vi "URG-04LX-UG01 Start Acquisition.vi"(8 "VISA Refnum in 2":refnum<visa-resource-name>, 10 "Acquisition Parameters":T1={"Starting Step"=0, "Ending Step"=0, "Cluster Count"=0, "Scan Interval"=0, "Number of Scans"=0, "Measurement Type"=enum."MS"}, 11 "error in (no error)":errorcluster) -> (0 "VISA Refnum in":refnum<visa-resource-name>, 2 "Acquisition Parameters":T1={"Starting Step"=0, "Ending Step"=0, "Cluster Count"=0, "Scan Interval"=0, "Number of Scans"=0, "Measurement Type"=enum."MS"}, 3 "error out":errorcluster)   [LabVIEW 2018]
doc: "Begins an acquisition task with the URG-04LX-UG01 based upon the specified <b>Acquisition Parameters</b>."
uses:
  Type Definitions/Acquisition Parameters.ctl
  Type Definitions/Measurement Type.ctl
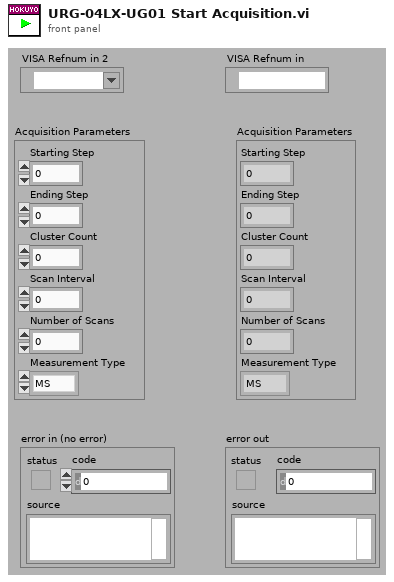
[diagram p1: front panel]
types:
  T1 = typedef "Acquisition Parameters.ctl" = cluster{"Starting Step":i32, "Ending Step":i32, "Cluster Count":i32, "Scan Interval":i32, "Number of Scans":i32, "Measurement Type":T2}
  T2 = typedef "Measurement Type.ctl" = enum16{"MD", "MS"}
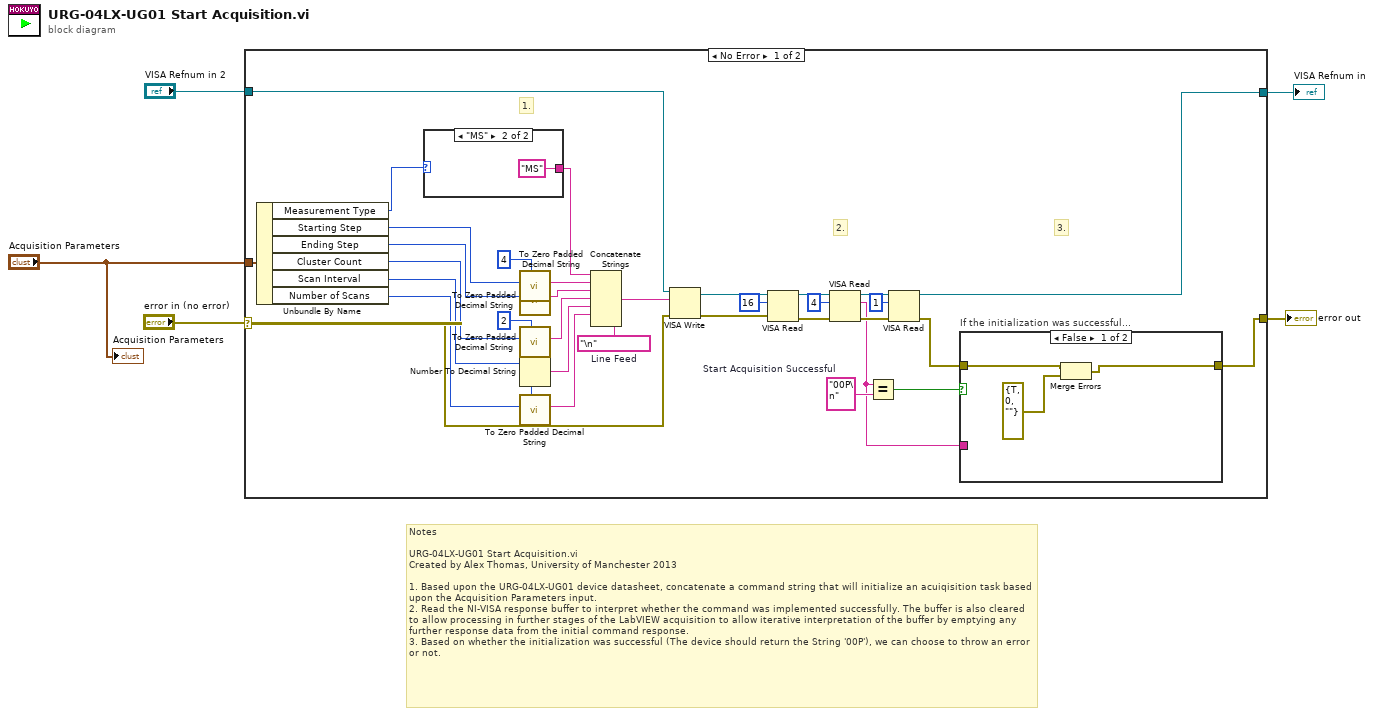
[diagram p0: block diagram]
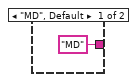
[diagram p3: hidden frame]
diagram:
  # "Notes\n\nURG-04LX-UG01 Start Acquisition.vi\nCreated by Alex Thomas, University of Manchester 2013\n\n1. Based upon the URG-04LX-UG01 device datasheet, concatenate a command string that will initialize an acuiqisition task based upon the Acquisition Parameters input. \n2. Read the NI-VISA response buffer to interpret whether the command was implemented successfully. The buffer is also cleared to allow processing in further stages of the LabVIEW acquisition to allow iterative interpretation of the buffer by emptying any further response data from the initial command response.\n3. Based on whether the initialization was successful (The device should return the String '00P'), we can choose to throw an error or not."
  n1 = case shown="No Error" "error in (no error)" {
    selector: "error in (no error)" -> [w22 w47]
    tunnel: [w9 w47] -> w2
    tunnel: "Acquisition Parameters" -> [w32 _]
    tunnel: "VISA Refnum in 2" -> [w23 w46]
    tunnel: [w11 w46] -> w5
    frame No Error {
      w8 = "00P\n"  # Start Acquisition Successful
      w25 = "\n"  # Line Feed
      w34 = 2 ("Required Padding Width")
      w38 = 4 ("Required Padding Width")
      # "3."
      # "2."
      # "1."
      n2 = Unbundle By Name(w32) -> ("Measurement Type"=w21:T2, "Starting Step"=w31:i32, "Ending Step"=w30:i32, "Cluster Count"=w29:i32, "Scan Interval"=w28:i32, "Number of Scans"=w27:i32)
      n3 = case shown="\"MS\"" w21 {
        tunnel: ["MD" "MS"] -> w26
        frame "MD", Default {
        }
        frame "MS" {
        }
      }
      n4 = call "To Zero Padded Decimal String.vi"("Required Padding Width"=w38, "Number"=w31) -> ("Padded Number"=w39:string)  [unwired: 9 in]
      n5 = call "To Zero Padded Decimal String.vi"("Required Padding Width"=w38, "Number"=w30) -> ("Padded Number"=w37:string)  [unwired: 9 in]
      n6 = call "To Zero Padded Decimal String.vi"("Required Padding Width"=w34, "Number"=w29) -> ("Padded Number"=w36:string)  [unwired: 9 in]
      n7 = Number To Decimal String(number=w28) -> (decimal integer string=w35:string)  [unwired: 1 in]
      n8 = call "To Zero Padded Decimal String.vi"("Required Padding Width"=w34, "Number"=w27) -> ("Padded Number"=w33:string)  [unwired: 9 in]
      n9 = Concatenate Strings(w26, w39, w37, w36, w35, w33, w25) -> (w24:string)
      n10 = VISA Write(VISA resource name=w23, write buffer=w24, error in (no error)=w22) -> (VISA resource name out=w15:refnum<visa-resource-name>, error out=w14:errorcluster)  [unwired: 1 out]
      n11 = VISA Read(VISA resource name=w15, byte count=u32 16, error in (no error)=w14) -> (VISA resource name out=w13:refnum<visa-resource-name>, error out=w12:errorcluster)  [unwired: 2 out]
      n12 = VISA Read(VISA resource name=w13, byte count=u32 4, error in (no error)=w12) -> (VISA resource name out=w17:refnum<visa-resource-name>, read buffer=w6:string, error out=w16:errorcluster)  [unwired: 1 out]
      n13 = Equal?(x=w6, y=w8) -> (x = y?=w10:bool)
      n14 = VISA Read(VISA resource name=w17, byte count=u32 1, error in (no error)=w16) -> (VISA resource name out=w11:refnum<visa-resource-name>, error out=w7:errorcluster)  [unwired: 2 out]
      n15 = case "If the initialization was successful..." shown="False" w10 {
        tunnel: [w41 w43] -> w9
        tunnel: w7 -> [w42 w43]
        tunnel: w6 -> [_ _]
        frame False {
          n16 = Merge Errors(w42, errorcluster {"status"=TRUE, "code"=0, "source"=""} ("error in")) -> (w41:errorcluster)
        }
        frame True {
        }
      }
    }
    frame Error {
    }
  }
  "VISA Refnum in" <- w5
  "error out" <- w2
  "Acquisition Parameters" <- "Acquisition Parameters"
